vi "Power Min Read Array.vi"(8 "error in":errorcluster, 11 "Power Supply In":refnum<class "Power Supply.lvclass">) -> (0 "error out":errorcluster, 1 "Changed or First Call?":bool, 2 "Power Min SP":dbl[](array[numeric]), 3 "Power Supply Out":refnum<class "Power Supply.lvclass">)   [LabVIEW 2023, in "Power Supply.lvclass"]
uses:
  Power Supply.lvclass
  Low Level Capabilities/Power/Power Limit/Power Limit.lvclass
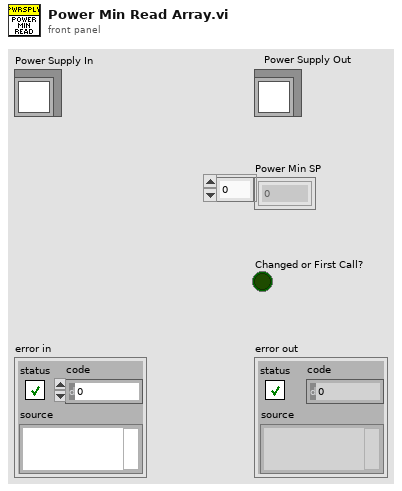
[diagram p1: front panel]
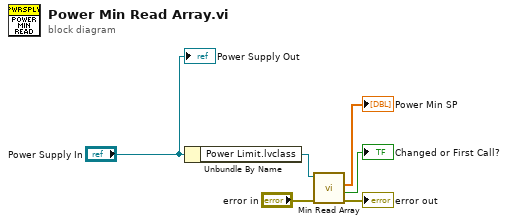
[diagram p0: block diagram]
diagram:
  n1 = Unbundle By Name("Power Supply In") -> ("Power Limit.lvclass"=w5:refnum<class "Power Limit.lvclass">)
  n2 = call-dynamic "Min Read Array.vi"("error in"="error in", "Min Power Limit in"=w5) -> ("error out"=→"error out":errorcluster, "Changed or First Call?"=→"Changed or First Call?":bool, "Power Min SP"=→"Power Min SP":dbl[])  [unwired: 6 in, 1 out]
  "Power Supply Out" <- "Power Supply In"
